vi "Test Resolve Relative.vi"() -> ()   [LabVIEW 2020]
uses:
  stream/URI/URI.lvclass
panel:
  out "Failures":T1(array[cluster])
  out "Result":bool
  in  "Base URI String":string="http://a/b/c/d;p?q"
  in  "Values":cluster{"URI":string, "Correct":string}[](array[cluster])=[{"URI"="g:h", "Correct"="g:h"}, {"URI"="g", "Correct"="http://a/b/c/g"}, {"URI"="./g", "Correct"="http://a/b/c/g"}, {"URI"="g/", "Correct"="http://a/b/c/g/"}, {"URI"="/g", "Correct"="http://a/g"}, {"URI"="//g", "Correct"="http://g"}, {"URI"="?y", "Correct"="http://a/b/c/d;p?y"}, {"URI"="g?y", "Correct"="http://a/b/c/g?y"}, {"URI"="#s", "Correct"="http://a/b/c/d;p?q#s"}, {"URI"="g#s", "Correct"="http://a/b/c/g#s"}, {"URI"="g?y#s", "Correct"="http://a/b/c/g?y#s"}, {"URI"=";x", "Correct"="http://a/b/c/;x"}, {"URI"="g;x", "Correct"="http://a/b/c/g;x"}, {"URI"="g;x?y#s", "Correct"="http://a/b/c/g;x?y#s"}, {"URI"="", "Correct"="http://a/b/c/d;p?q"}, {"URI"=".", "Correct"="http://a/b/c/"}, {"URI"="./", "Correct"="http://a/b/c/"}, {"URI"="..", "Correct"="http://a/b/"}, {"URI"="../", "Correct"="http://a/b/"}, {"URI"="../g", "Correct"="http://a/b/g"}, {"URI"="../..", "Correct"="http://a/"}, {"URI"="../../", "Correct"="http://a/"}, {"URI"="../../g", "Correct"="http://a/g"}]
  # "Correct Result"
  # "Parse"
  # "Parsed As"
  # "Result"
  # "Should Be"
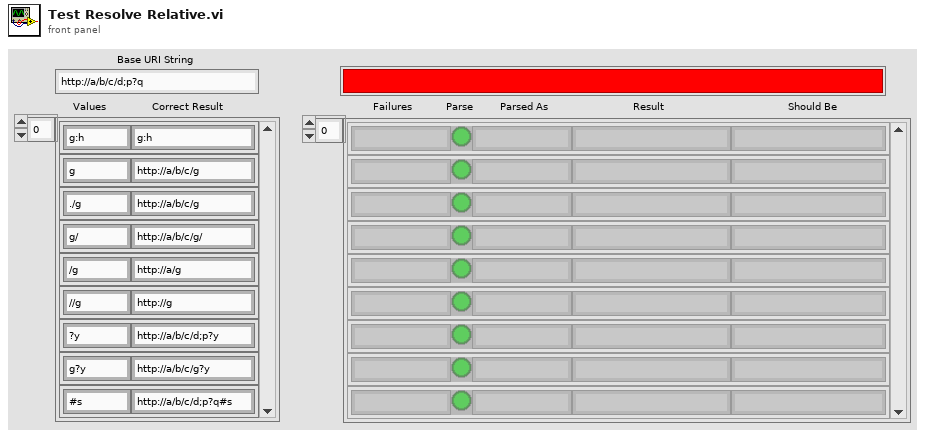
[diagram p1: front panel]
types:
  T1 = cluster{"URI":string, bool, "URI String":string, "URI String":string, "Correct":string}[]
  T2 = cluster{"URI":string, bool, "URI String":string, "URI String":string, "Correct":string}
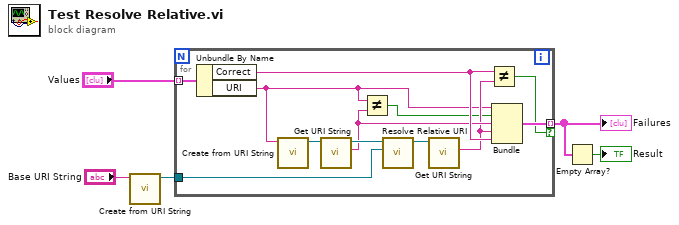
[diagram p0: block diagram]
diagram:
  n1 = call "Create from URI String.vi"("URI String"="Base URI String") -> ("URI out"=w4:refnum<class "URI.lvclass">)  [unwired: 9 in, 1 out]
  n2 = for {
    tunnel: w4 -> [w16]
    tunnel: "Values" -> [w17] mode=indexing
    tunnel: [w13] -> w2 mode=indexing if=w12
    n3 = Unbundle By Name(w17) -> ("Correct"=w14:string, "URI"=w6:string)
    n4 = call "Create from URI String.vi"("URI String"=w6) -> ("URI out"=w11:refnum<class "URI.lvclass">)  [unwired: 9 in, 1 out]
    n5 = call "Get URI String.vi"("URI in"=w11) -> ("URI String"=w9:string, "URI out"=w10:refnum<class "URI.lvclass">)  [unwired: 8 in, 1 out]
    n6 = Not Equal?(x=w6, y=w9) -> (x != y?=w7:bool)
    n7 = call "Resolve Relative URI.vi"("Base URI"=w16, "URI in"=w10) -> ("URI out"=w15:refnum<class "URI.lvclass">)  [unwired: 8 in, 1 out]
    n8 = call "Get URI String.vi"("URI in"=w15) -> ("URI String"=w8:string)  [unwired: 8 in, 2 out]
    n9 = Not Equal?(x=w14, y=w8) -> (x != y?=w12:bool)
    n10 = Bundle("URI"=w6, w7, "URI String"=w9, "URI String"=w8, "Correct"=w14) -> (w13:T2)  [unwired: 1 in]
  }
  "Failures" <- w2
  n11 = Empty Array?(array=w2) -> (empty?=→"Result":bool)
